vi "Add Tx UDP VLs and UDPs.vi"(8 "error in":errorcluster, 10 "Tx UDP configuration":T7(array[cluster]) {"sapPorts"."Parameters"."Parameter"."encoding" items=["BNR", "BCD", "Discrete", "Signed_32", "Signed_64", "Float_32", "Float_64", "Opaque"]; "commPorts"."Parameters"."Parameter"."encoding" items=["BNR", "BCD", "Discrete", "Signed_32", "Signed_64", "Float_32", "Float_64", "Opaque"]; "tx_udp_setup"."NumOfSubVl" format="%.0b"; "tx_udp_setup"."NetSelect" items=["FDX_TX_FRAME_DLY_A", "FDX_TX_FRAME_DLY_B", "FDX_TX_FRAME_BOTH", "FDX_TX_FRAME_ONLY_A", "FDX_TX_FRAME_ONLY_B"]}, 11 "Tx UDP ref":T8 format="%.0x") -> (0 "error out":errorcluster, 3 "Tx UDP ref out":T8 format="%.0x")   [LabVIEW 2020, in "AIM ARINC 664 Scripting.lvlib"]
doc: "Add the UDP VLs, UDP ports and parameters based on the Tx UDP configuration."
uses:
  AIM ARINC 664 Scripting.lvlib
  <vilib>/NI VeriStand/Custom Device API/Custom Device API.lvlib
  Constants.vi
  <vilib>/NI VeriStand/Custom Device API/Custom Device Channel Type.ctl
  <vilib>/NI VeriStand/Custom Device API/Custom Device Channel.ctl
  <instrlib>/AIM GmbH/_AIM 664/_controls/comm_udp_tx.ctl
  <instrlib>/AIM GmbH/_AIM 664/AIM664LV.lvlib
  <instrlib>/AIM GmbH/_AIM 664/_controls/comm_config_vl_tx.ctl
  Shared/Encoding (Arinc664).ctl
  Import/_typedefs/frame_parameter_definition.ctl
  Import/AIM ARINC 664 Import.lvlib
  <vilib>/NI VeriStand/Custom Device API/Set Item Property (String).vi
  <vilib>/NI VeriStand/Custom Device API/Custom Device Item Ref.ctl
  Import/_typedefs/tx_udp_setup.ctl
  Import/_typedefs/frame_parameter.ctl
  Import/_typedefs/port_tx_udp_comm.ctl
  Import/_typedefs/port_tx_udp_sap.ctl
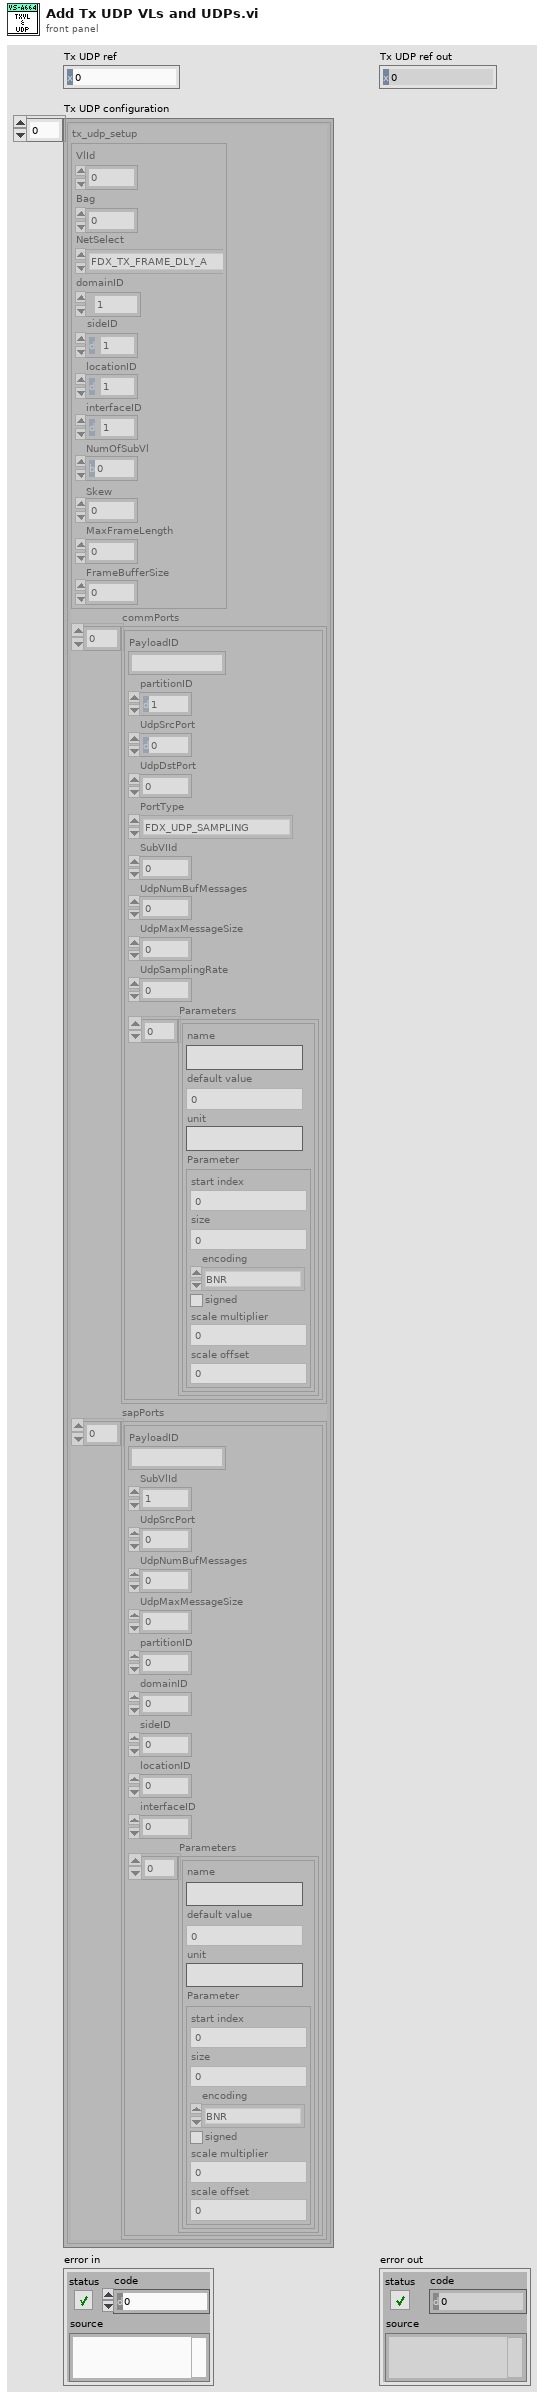
[diagram p1: front panel]
types:
  T1 = typedef "AIM ARINC 664 Import.lvlib/tx_udp_setup.ctl" = cluster{"VlId":i32, "Bag":i32, "NetSelect":u32, "domainID":u8, "sideID":u8, "locationID":u8, "interfaceID":u8, "NumOfSubVl":u16, "Skew":u32, "MaxFrameLength":u32, "FrameBufferSize":u32}
  T2 = typedef "AIM ARINC 664 Import.lvlib/port_tx_udp_comm.ctl" = cluster{"PayloadID":string, "partitionID":u8, "UdpSrcPort":u16, "UdpDstPort":u16, "PortType":enum16{"FDX_UDP_SAMPLING", "FDX_UDP_QUEUING"}, "SubVIId":u32, "UdpNumBufMessages":u32, "UdpMaxMessageSize":u32, "UdpSamplingRate":u32, "Parameters":T3[]}
  T3 = typedef "AIM ARINC 664 Import.lvlib/frame_parameter.ctl" = cluster{"name":string, "default value":dbl, "unit":string, "Parameter":T4}
  T4 = typedef "AIM ARINC 664 Import.lvlib/frame_parameter_definition.ctl" = cluster{"start index":i32, "size":i32, "encoding":T5, "signed":bool, "scale multiplier":dbl, "scale offset":dbl}
  T5 = typedef "Encoding (Arinc664).ctl" = u16
  T6 = typedef "AIM ARINC 664 Import.lvlib/port_tx_udp_sap.ctl" = cluster{"PayloadID":string, "SubVlId":u8, "UdpSrcPort":u16, "UdpNumBufMessages":u32, "UdpMaxMessageSize":u32, "partitionID":u8, "domainID":u8, "sideID":u8, "locationID":u8, "interfaceID":u8, "Parameters":T3[]}
  T7 = cluster{"tx_udp_setup":T1, "commPorts":T2[], "sapPorts":T6[]}[]
  T8 = typedef "Custom Device API.lvlib/Custom Device Item Ref.ctl" = u64
  T9 = typedef "AIM664LV.lvlib/comm_config_vl_tx.ctl" = cluster{"VlId":u16, "NumOfSubVl":u16, "rate ms [Bag]":u32, "domainID":u8, "sideID":u8, "locationID":u8, "interfaceID":u8, "NetSelect":u32, "Skew":u32, "MaxFrameLength":u32, "FrameBufferSize":u32}
  T10 = typedef "AIM664LV.lvlib/comm_udp_tx.ctl" = cluster{"PortType":enum16{"FDX_UDP_SAMPLING", "FDX_UDP_QUEUING"}, "partitionID":u8, "SubVlId":u8, "UdpSrcPort":u16, "UdpDstPort":u16, "SampleRateMs":dbl, "UdpNumBufMessages":u32, "UdpMaxMessageSize":u32}
  T11 = typedef "Custom Device API.lvlib/Custom Device Channel Type.ctl" = enum16{"Input", "Output"}
  T12 = typedef "Custom Device API.lvlib/Custom Device Channel.ctl" = cluster{"Type":T11, "Units":string, "Default Value":dbl, "Faultable":bool, "Scalable":bool}
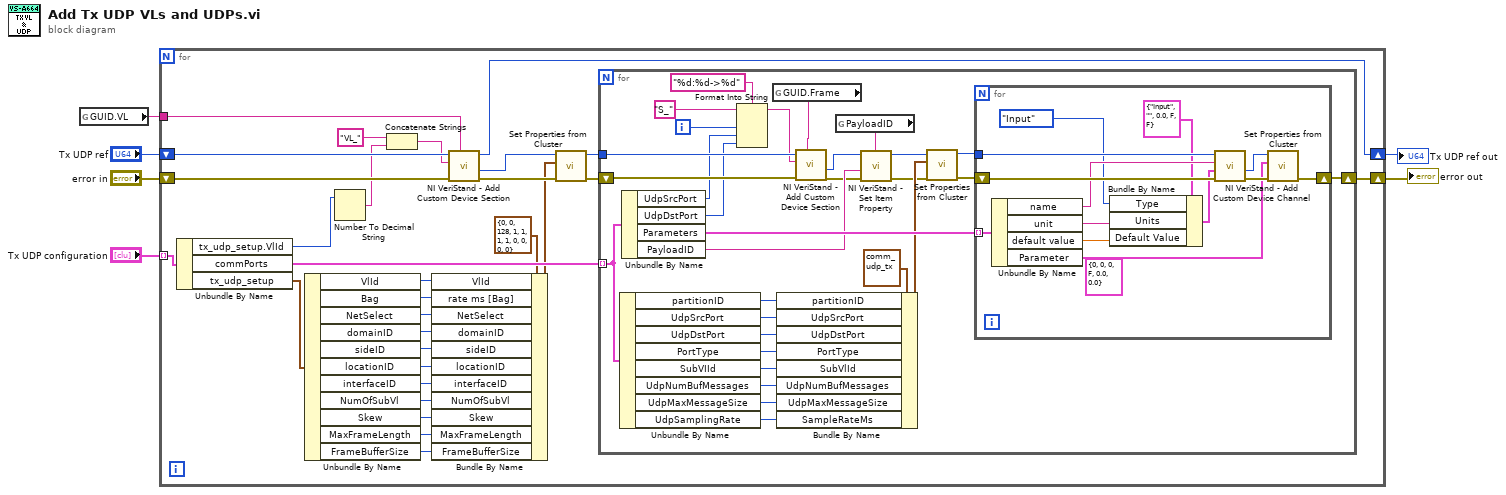
[diagram p0: block diagram]
diagram:
  n1 = global read "Constants.vi" "GUID.VL"() -> (w2:string)
  n2 = for {
    tunnel: "Tx UDP configuration" -> [w25] mode=indexing
    shift-right: [w26] -> w1
    shift-left: "Tx UDP ref" -> [w35]
    shift-right: [w33] -> w3
    shift-left: "error in" -> [w34]
    tunnel: w2 -> [w27]
    n3 = Unbundle By Name(w25) -> ("tx_udp_setup.VlId"=w29:i32, "commPorts"=w28:T2[], "tx_udp_setup"=w19:T1)
    n4 = Unbundle By Name(w19) -> ("VlId"=w17:i32, "Bag"=w16:i32, "NetSelect"=w15:u32, "domainID"=w14:u8, "sideID"=w13:u8, "locationID"=w12:u8, "interfaceID"=w11:u8, "NumOfSubVl"=w10:u16, "Skew"=w9:u32, "MaxFrameLength"=w8:u32, "FrameBufferSize"=w7:u32)
    n5 = Number To Decimal String(number=w29) -> (decimal integer string=w31:string)  [unwired: 1 in]
    n6 = Concatenate Strings("VL_" ("string"), w31) -> (w30:string)
    n7 = Bundle By Name(cluster=T9 {"VlId"=0, "NumOfSubVl"=0, "rate ms [Bag]"=128, "domainID"=1, "sideID"=1, "locationID"=1, "interfaceID"=1, "NetSelect"=0, "Skew"=0, "MaxFrameLength"=0, "FrameBufferSize"=0} ("CommPort Config"), "VlId"=w17, "rate ms [Bag]"=w16, "NetSelect"=w15, "domainID"=w14, "sideID"=w13, "locationID"=w12, "interfaceID"=w11, "NumOfSubVl"=w10, "Skew"=w9, "MaxFrameLength"=w8, "FrameBufferSize"=w7) -> (w18:T9)
    n8 = call <vilib>:"NI VeriStand - Add Custom Device Section.vi"("GUID (Default Section)"=w27, "error in (no error)"=w34, "Section Name"=w30, "Parent Ref in"=w35) -> ("error out"=w24:errorcluster, "Section Ptr"=w22:T8, "Parent Ref out"=w26:T8)  [unwired: 4 in, 1 out]
    n9 = call "Set Properties from Cluster.vi"("error in"=w24, "Variant Cluster"=w18, "item ref in"=w22) -> ("error out"=w23:errorcluster, "item ref out"=w21:T8)  [unwired: 7 in]
    n10 = for {
      shift-right: [w62] -> w33
      shift-left: w23 -> [w64]
      tunnel: w28 -> [w52] mode=indexing
      tunnel: w21 -> [w65]
      i -> [w60]
      n11 = Unbundle By Name(w52) -> ("partitionID"=w51:u8, "UdpSrcPort"=w50:u16, "UdpDstPort"=w49:u16, "PortType"=w48:enum16{"FDX_UDP_SAMPLING", "FDX_UDP_QUEUING"}, "SubVIId"=w47:u32, "UdpNumBufMessages"=w46:u32, "UdpMaxMessageSize"=w45:u32, "UdpSamplingRate"=w44:u32)
      n12 = Unbundle By Name(w52) -> ("UdpSrcPort"=w58:u16, "UdpDstPort"=w57:u16, "Parameters"=w63:T3[], "PayloadID"=w41:string)
      n13 = Format Into String(format string="%d:%d->%d", initial string="S_" ("string"), w60, w58, w57) -> (resulting string=w56:string)  [unwired: 1 in, 1 out]
      n14 = global read "Constants.vi" "GUID.Frame"() -> (w36:string)
      n15 = Bundle By Name(cluster=T10 {"PortType"=enum."FDX_UDP_SAMPLING", "partitionID"=0, "SubVlId"=1, "UdpSrcPort"=0, "UdpDstPort"=0, "SampleRateMs"=128.0, "UdpNumBufMessages"=0, "UdpMaxMessageSize"=0} ("commPort config"), "partitionID"=w51, "UdpSrcPort"=w50, "UdpDstPort"=w49, "PortType"=w48, "SubVlId"=w47, "UdpNumBufMessages"=w46, "UdpMaxMessageSize"=w45, "SampleRateMs"=w44) -> (w43:T10)
      n16 = call <vilib>:"NI VeriStand - Add Custom Device Section.vi"("GUID (Default Section)"=w36, "error in (no error)"=w64, "Section Name"=w56, "Parent Ref in"=w65) -> ("error out"=w40:errorcluster, "Section Ptr"=w38:T8)  [unwired: 4 in, 2 out]
      n17 = global read "Constants.vi" "PayloadID"() -> (w37:string)
      n18 = call-poly <vilib>:"NI VeriStand - Set Item Property.vi"("error in (no error)"=w40, "Value"=w41, "Property Name"=w37, "Item Ref in"=w38) -> ("error out"=w39:errorcluster, "Item Ref out"=w42:T8)  [unwired: 5 in, 1 out]
      n19 = call "Set Properties from Cluster.vi"("error in"=w39, "Variant Cluster"=w43, "item ref in"=w42) -> ("error out"=w54:errorcluster, "item ref out"=w55:T8)  [unwired: 7 in]
      n20 = for {
        tunnel: w55 -> [w78]
        tunnel: w63 -> [w76] mode=indexing
        shift-right: [w69] -> w62
        shift-left: w54 -> [w77]
        (unwired) T4 {"start index"=0, "size"=0, "encoding"=0, "signed"=FALSE, "scale multiplier"=0.0, "scale offset"=0.0} ("Parameter")
        n21 = Unbundle By Name(w76) -> ("name"=w75:string, "unit"=w72:string, "default value"=w71:dbl, "Parameter"=w68:T4)
        n22 = Bundle By Name(cluster=T12 {"Type"=enum."Input", "Units"="", "Default Value"=0.0, "Faultable"=FALSE, "Scalable"=FALSE} ("Channel"), "Type"=Custom_Device_Channel_Type."Input", "Units"=w72, "Default Value"=w71) -> (w73:T12)
        n23 = call <vilib>:"NI VeriStand - Add Custom Device Channel.vi"("error in (no error)"=w77, "Channel"=w73, "Channel Name"=w75, "Parent Ref in"=w78) -> ("error out"=w70:errorcluster, "Channel Ref"=w67:T8)  [unwired: 4 in, 2 out]
        n24 = call "Set Properties from Cluster.vi"("error in"=w70, "Variant Cluster"=w68, "item ref in"=w67) -> ("error out"=w69:errorcluster)  [unwired: 7 in, 1 out]
      }
    }
  }
  "Tx UDP ref out" <- w1
  "error out" <- w3
